vi "仪器参数设置.vi"(11 "氨氮仪器参数":T2) -> (3 "仪器参数设置输出":T1)   [LabVIEW 2016, in "斯坦道总磷.lvlib"]
uses:
  <vilib>/Utility/miscctls.llb/LVPointTypeDef.ctl
panel:
  in  "标样校准时间":timestamp
  in  "二次多项式系数":dbl
  in  "线性相关系数":dbl
  in  "测量信号值":dbl
  in  "测量检出限":dbl
  in  "曲线斜率":dbl
  in  "曲线截距":dbl
  in  "空白校准时间":timestamp
  in  "消解时长":dbl
  in  "消解温度":dbl
  in  "测量间隔":dbl
  in  "测量精度":dbl
  in  "测量量程":dbl
  in  "取消":bool
  in  "确定":bool
  # "仪器参数设置"
  # "总磷"
  # "监测参数"
  # "黑色框参数需要手动输入\n灰色框参数自动读取不需要手动输入"
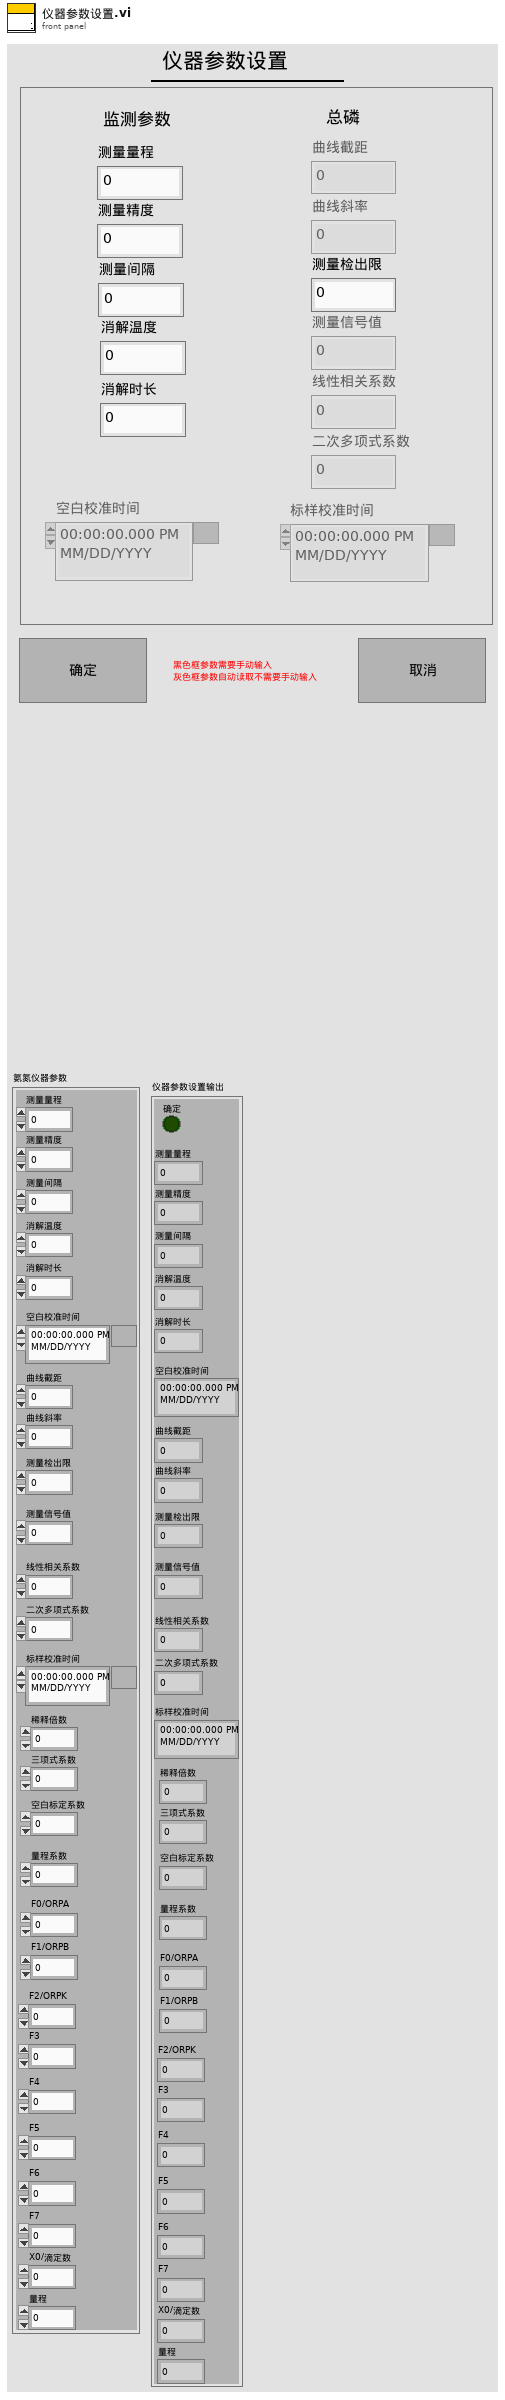
[diagram p1: front panel]
types:
  T1 = cluster{"确定":bool, "测量量程":dbl, "测量精度":dbl, "测量间隔":dbl, "消解温度":dbl, "消解时长":dbl, "空白校准时间":timestamp, "曲线截距":dbl, "曲线斜率":dbl, "测量检出限":dbl, "测量信号值":dbl, "线性相关系数":dbl, "二次多项式系数":dbl, "标样校准时间":timestamp, "稀释倍数":dbl, "三项式系数":dbl, "空白标定系数":dbl, "量程系数":dbl, "F0/ORPA":dbl, "F1/ORPB":dbl, "F2/ORPK":dbl, "F3":dbl, "F4":dbl, "F5":dbl, "F6":dbl, "F7":dbl, "X0/滴定数":dbl, "量程":dbl}
  T2 = cluster{"测量量程":dbl, "测量精度":dbl, "测量间隔":dbl, "消解温度":dbl, "消解时长":dbl, "空白校准时间":timestamp, "曲线截距":dbl, "曲线斜率":dbl, "测量检出限":dbl, "测量信号值":dbl, "线性相关系数":dbl, "二次多项式系数":dbl, "标样校准时间":timestamp, "稀释倍数":dbl, "三项式系数":dbl, "空白标定系数":dbl, "量程系数":dbl, "F0/ORPA":dbl, "F1/ORPB":dbl, "F2/ORPK":dbl, "F3":dbl, "F4":dbl, "F5":dbl, "F6":dbl, "F7":dbl, "X0/滴定数":dbl, "量程":dbl}
  T3 = typedef "LVPointTypeDef.ctl" = cluster{"Horizontal":i16, "Vertical":i16}
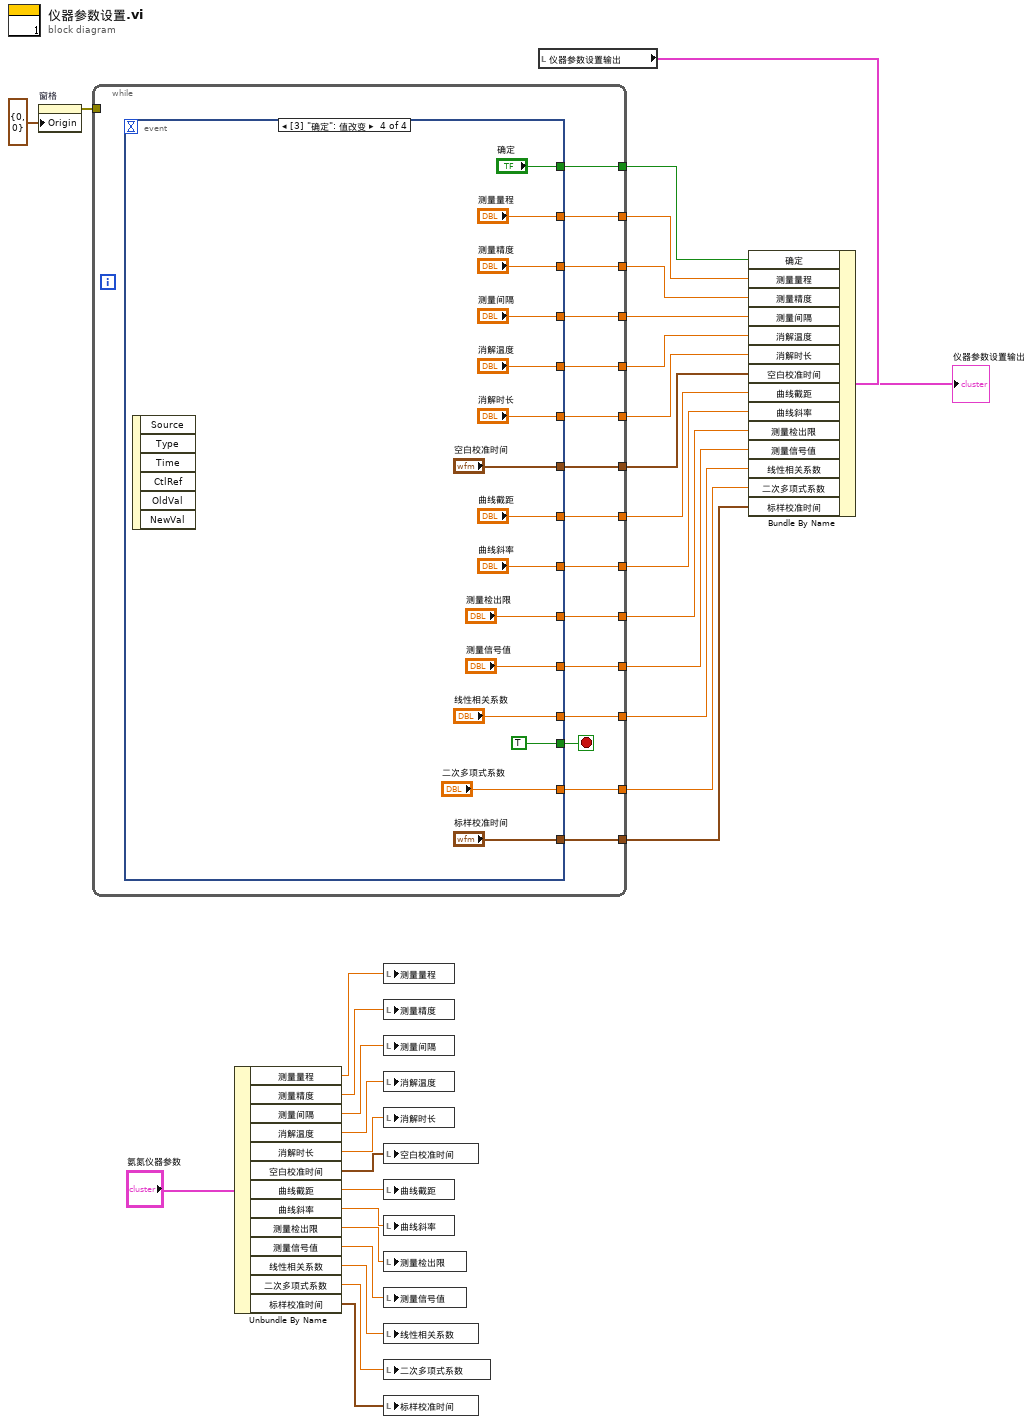
[diagram p0: block diagram]
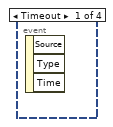
[diagram p2: hidden frame]
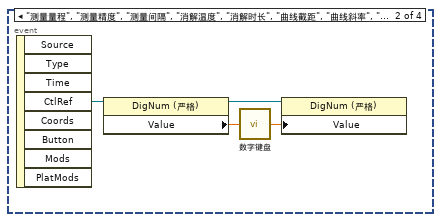
[diagram p3: hidden frame]
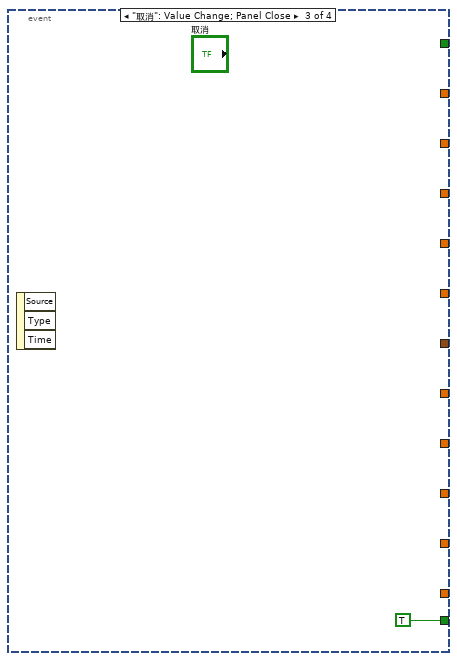
[diagram p4: hidden frame]
diagram:
  n1 = property on="窗格" class="Pane"("Origin"=T3 {"Horizontal"=0, "Vertical"=0} ("原点")) -> (error out=w31:errorcluster)  [unwired: 2 in, 1 out]
  n2 = while {
    tunnel: w31 -> [_]
    tunnel: [w46] -> w30
    tunnel: [w45] -> w28
    tunnel: [w44] -> w27
    tunnel: [w43] -> w26
    tunnel: [w42] -> w25
    tunnel: [w41] -> w24
    tunnel: [w40] -> w23
    tunnel: [w39] -> w22
    tunnel: [w38] -> w21
    tunnel: [w37] -> w20
    tunnel: [w36] -> w19
    tunnel: [w35] -> w18
    tunnel: [w34] -> w17
    tunnel: [w33] -> w16
    stop <- w47 stop-if-true
    n3 = event shown="[3] \"确定\": 值改变" {
      selector: _ -> [_ _ _ _]
      dyn-events: _ -> [_ _ _ _]
      timeout: _ -> [_ _ _ _]
      tunnel: [_ _ TRUE TRUE] -> w47
      tunnel: [_ _ _ "确定"] -> w46
      tunnel: [_ _ _ "标样校准时间"] -> w45
      tunnel: [_ _ _ "二次多项式系数"] -> w44
      tunnel: [_ _ _ "线性相关系数"] -> w43
      tunnel: [_ _ _ "测量信号值"] -> w42
      tunnel: [_ _ _ "测量检出限"] -> w41
      tunnel: [_ _ _ "曲线斜率"] -> w40
      tunnel: [_ _ _ "曲线截距"] -> w39
      tunnel: [_ _ _ "空白校准时间"] -> w38
      tunnel: [_ _ _ "消解时长"] -> w37
      tunnel: [_ _ _ "消解温度"] -> w36
      tunnel: [_ _ _ "测量间隔"] -> w35
      tunnel: [_ _ _ "测量精度"] -> w34
      tunnel: [_ _ _ "测量量程"] -> w33
      event Timeout {
        n4 = event-data() -> ()  [unwired: 1 in, 3 out]
      }
      event "测量量程", "测量精度", "测量间隔", "消解温度", "消解时长", "曲线截距", "曲线斜率", "测量检出限", "测量信号值", "线性相关系数", "二次多项式系数": Mouse Down {
        n5 = event-data() -> ("CtlRef"=w48:refnum<vi>)  [unwired: 1 in, 7 out]
        n6 = property class="DigNum (严格)"(reference=w48) -> (reference out=w50:refnum<vi>, "Value"=w51:dbl)  [unwired: 1 in, 1 out]
        n7 = call "数字键盘.vi"("OldNumber"=w51) -> ("NewNumber"=w49:dbl)
        n8 = property class="DigNum (严格)"(reference=w50, "Value"=w49) -> ()  [unwired: 1 in, 2 out]
      }
      event "取消": Value Change; Panel Close {
        n9 = event-data() -> ()  [unwired: 1 in, 3 out]
      }
      event "确定": Value Change {
        n10 = event-data() -> ()  [unwired: 1 in, 6 out]
      }
    }
  }
  n11 = Unbundle By Name("氨氮仪器参数") -> ("测量量程"=w15:dbl, "测量精度"=w14:dbl, "测量间隔"=w13:dbl, "消解温度"=w12:dbl, "消解时长"=w11:dbl, "空白校准时间"=w10:timestamp, "曲线截距"=w9:dbl, "曲线斜率"=w8:dbl, "测量检出限"=w7:dbl, "测量信号值"=w6:dbl, "线性相关系数"=w5:dbl, "二次多项式系数"=w4:dbl, "标样校准时间"=w3:timestamp)
  n12 = local write "测量量程"(w15) -> ()
  n13 = local write "测量精度"(w14) -> ()
  n14 = local write "测量间隔"(w13) -> ()
  n15 = local write "消解温度"(w12) -> ()
  n16 = local write "消解时长"(w11) -> ()
  n17 = local write "空白校准时间"(w10) -> ()
  n18 = local write "曲线截距"(w9) -> ()
  n19 = local write "曲线斜率"(w8) -> ()
  n20 = local write "测量检出限"(w7) -> ()
  n21 = local write "测量信号值"(w6) -> ()
  n22 = local write "线性相关系数"(w5) -> ()
  n23 = local write "二次多项式系数"(w4) -> ()
  n24 = local write "标样校准时间"(w3) -> ()
  n25 = local read "仪器参数设置输出"() -> (w29:T1)
  n26 = Bundle By Name(cluster=w29, "确定"=w30, "测量量程"=w16, "测量精度"=w17, "测量间隔"=w18, "消解温度"=w19, "消解时长"=w20, "空白校准时间"=w21, "曲线截距"=w22, "曲线斜率"=w23, "测量检出限"=w24, "测量信号值"=w25, "线性相关系数"=w26, "二次多项式系数"=w27, "标样校准时间"=w28) -> (→"仪器参数设置输出":T1)
